vi "client.vi"() -> ()   [LabVIEW 2018]
uses:
  <vilib>/userdefined/High Color/IMAQdx.ctl
  <vilib>/httpClient/POSTBuffer.vi
  <vilib>/vision/driver/NI_Vision_Acquisition_Software.lvlib
  <vilib>/addons/_JKI.lib/Serialization/JSON/JKI JSON Serialization.lvlib
  <vilib>/httpClient/LabVIEWHTTPClient.lvlib
panel:
  out "String":string
  out "доступ есть/нет":bool
  out "Array":cluster{"photo":string}[](array[cluster])
  out "headers":string
  out "String 2":string
  out "base64":string
  out "string":string
  in  "сделать фото":bool
  out "error out 4":errorcluster
  out "error out 3":errorcluster
  out "error out 2":errorcluster
  in  "stop":bool
  out "Image":T1(plugin-control)
  out "error out":errorcluster
  in  "Session In":T2
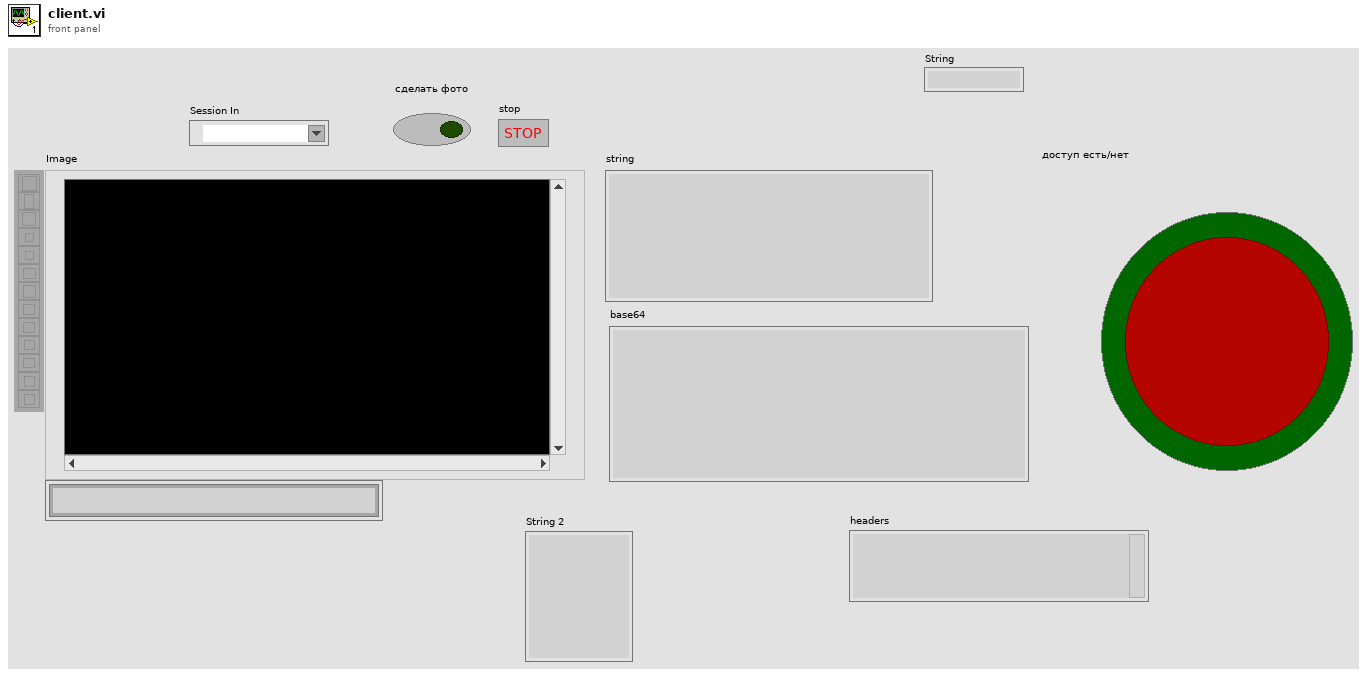
[diagram p1: front panel]
types:
  T1 = typedef "IMAQ Image.ctl" = refnum<image>
  T2 = typedef "IMAQdx.ctl" = refnum<k21>
  T3 = typedef "LabVIEWHTTPClient.lvlib/ClientHandle.ctl" = refnum<k1>
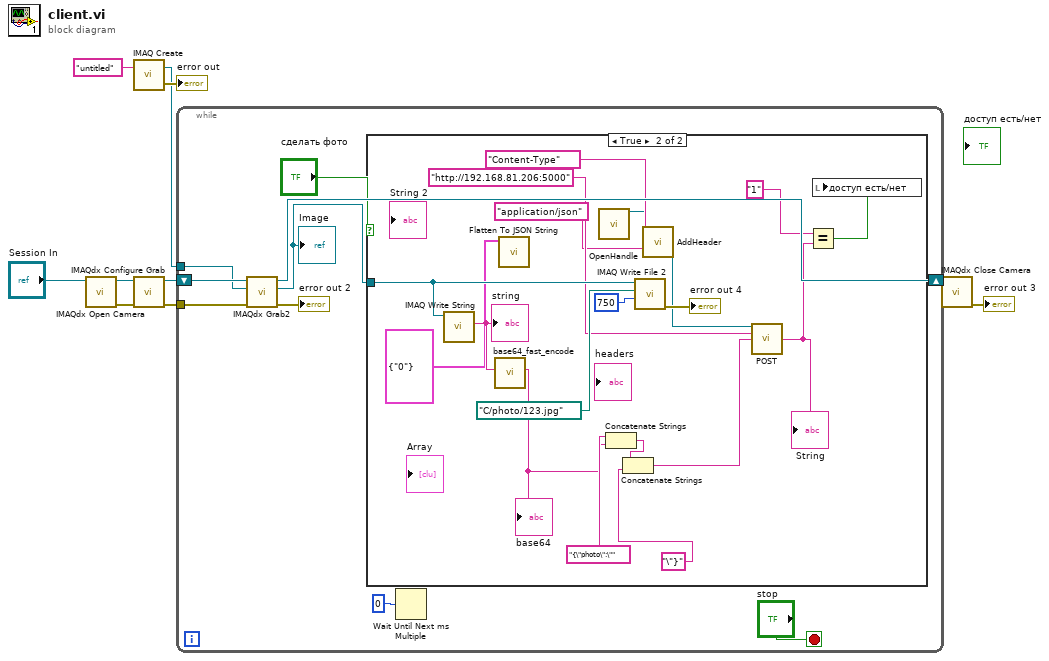
[diagram p0: block diagram]
diagram:
  n1 = call <vilib>:"IMAQdx Open Camera.vi"("Session In"="Session In") -> ("error out"=w3:errorcluster, "Session Out"=w2:T2)  [unwired: 9 in]
  n2 = call "IMAQ Create"("Image Name"="untitled") -> ("New Image"=w5:T1, "error out"=→"error out":errorcluster)  [unwired: 4 in]
  n3 = call <vilib>:"IMAQdx Configure Grab.vi"("error in"=w3, "Session In"=w2) -> ("error out"=w9:errorcluster, "Session Out"=w4:T2)  [unwired: 8 in]
  n4 = while {
    tunnel: w5 -> [w18]
    shift-right: [w17] -> w8
    shift-left: w4 -> [w19]
    tunnel: w9 -> [w15]
    stop <- "stop" stop-if-true
    n5 = call <vilib>:"IMAQdx Grab2.vi"("error in"=w15, "Image In"=w18, "Session In"=w19) -> ("error out"=→"error out 2":errorcluster, "Image Out"=w12:T1, "Session Out"=w17:T2)  [unwired: 5 in, 1 out]
    "Image" <- w12
    n6 = case shown="True" "сделать фото" {
      tunnel: w12 -> [_ w36]
      frame False {
      }
      frame True {
        n7 = call-poly "IMAQ Write String"("Image"=w36) -> ("FileString"=w35:string)  [unwired: 8 in, 2 out]
        "string" <- w35
        n8 = call "base64_fast_encode.vi"("string in (not encoded)"=w35) -> ("string out (base64-encoded)"=w26:string)  [unwired: 9 in, 1 out]
        "base64" <- w26
        n9 = call <vilib>:"Flatten To JSON String.vi"("Variant"=cluster{"photo":string} {"photo"="0"}) -> ()  [unwired: 9 in, 2 out]
        n10 = call <vilib>:"OpenHandle.vi"() -> ("client handle out"=w28:T3)  [unwired: 14 in, 1 out]
        n11 = Concatenate Strings("{\"photo\":\"", w26) -> (w25:string)
        n12 = Concatenate Strings(w25, "\"}") -> (w23:string)
        n13 = call-poly "IMAQ Write File 2"("Image Quality"=u32 750, "File Path"=path "C:/photo/123.jpg", "Image"=w36) -> ("error out"=→"error out 4":errorcluster)  [unwired: 7 in, 1 out]
        n14 = call <vilib>:"AddHeader.vi"("client handle"=w28, "header"="Content-Type", "value"="application/json") -> ("client handle out"=w29:T3)  [unwired: 11 in, 1 out]
        n15 = call-poly <vilib>:"POST.vi"("client handle"=w29, "url"="http://192.168.81.206:5000", "buffer"=w23) -> ("body"=w22:string)  [unwired: 9 in, 3 out]
        "String" <- w22
        n16 = Equal?(x="1", y=w22) -> (x = y?=w20:bool)
        n17 = local write "доступ есть/нет"(w20) -> ()
      }
    }
    n18 = Wait Until Next ms Multiple(millisecond multiple=u32 0) -> ()  [unwired: 1 out]
  }
  n19 = call <vilib>:"IMAQdx Close Camera.vi"("Session In"=w8) -> ("error out"=→"error out 3":errorcluster)  [unwired: 10 in]
